vi "List-Modify Item Name(Keep ID).vi"(7 "Separate Sign":string="-", 9 "New Name":string, 11 "List in":refnum<vi>) -> (3 "List Out":refnum<vi>)   [LabVIEW 2022 SP3]
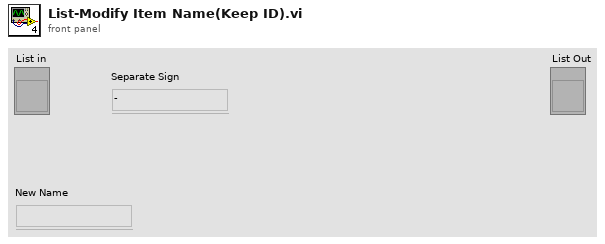
[diagram p1: front panel]
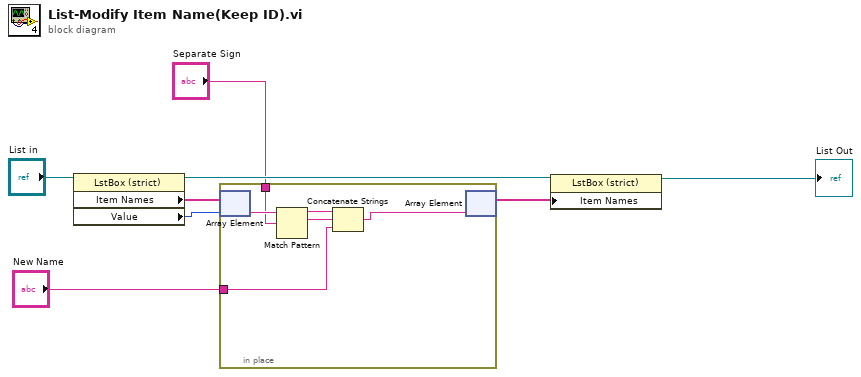
[diagram p0: block diagram]
diagram:
  n1 = property class="LstBox (strict)"(reference="List in") -> (reference out=w7:refnum<vi>, "Item Names"=w5:string[], "Value"=w4:i32)  [unwired: 1 in, 1 out]
  n2 = in-place {
    in-place-border: "Separate Sign" -> [w13]
    in-place-border: "New Name" -> [w10]
    n3 = in-place-array #1(w5, w4) -> (w14:string)
    n4 = Match Pattern(string=w14, regular expression=w13) -> (before substring=w12:string, match substring=w11:string)  [unwired: 1 in, 2 out]
    n5 = Concatenate Strings(w12, w11, w10) -> (w9:string)
    n6 = in-place-array #1(w9) -> (w3:string[])  [unwired: 1 out]
  }
  n7 = property class="LstBox (strict)"(reference=w7, "Item Names"=w3) -> (reference out=→"List Out":refnum<vi>)  [unwired: 1 in, 1 out]
